vi "lab1_byte_packet_transceiver.vi"() -> ()   [LabVIEW 2014]
uses:
  <vilib>/addons/Modulation/Analog/controls/Complex Data Waveform.ctl
  <vilib>/addons/Modulation/Analog/support/mod_Set Error Source.vi
  <vilib>/addons/Modulation/Digital/Support/Common/Validators/mod_AWGN Validate.vi
  <vilib>/addons/Modulation/Digital/Impairments/subVIs/mod_createSeeds.vi
  <vilib>/addons/Modulation/Digital/Support/Common/Validators/mod_Validate Samples Per Symbol.vi
  <vilib>/addons/Modulation/Analog/support/Validators/mod_Validate Complex Waveform.vi
  <vilib>/addons/Modulation/Analog/support/Validators/mod_WFErrorHandler.vi
  <vilib>/addons/Modulation/Digital/General/MT Generate PSK System Parameters(M).vi
  <vilib>/addons/Modulation/Digital/Support/Common/Validators/mod_Generate Filter Coefficients Validate.vi
  <vilib>/addons/Modulation/Digital/General/subVIs/mod_Generate Filter Coefficients.vi
  <vilib>/addons/Modulation/Digital/General/subVIs/mod_Generate Bits PN Sequence.vi
  <vilib>/Analysis/1siggen.llb/Gaussian White Noise (obs 90).vi
  <vilib>/addons/Modulation/niDMT.lvlib
  <vilib>/addons/Modulation/niAMT.lvlib
panel:
  out "packet counter":u32
  in  "Eb/N0 (10 dB)":dbl=10.0 format="%.2f"
  out "Constellation Graph":T1(graph)
  in  "filter length (symbols)":i32=8
  in  "filter parameter":dbl=0.5 format="%.2f"
  in  "pulse shaping filter (none)":T2(ring)
  in  "M-PSK (4)":i32=4
  in  "samples per symbol (16)":i32=16
  out "rx history":string
  out "tx history":string
  out "rx instant":string
  out "found?":bool
  out "byte length":u32
  in  "OK Button":bool
  in  "stop":bool
  out "size(s)":i32
  in  "tx instant":string
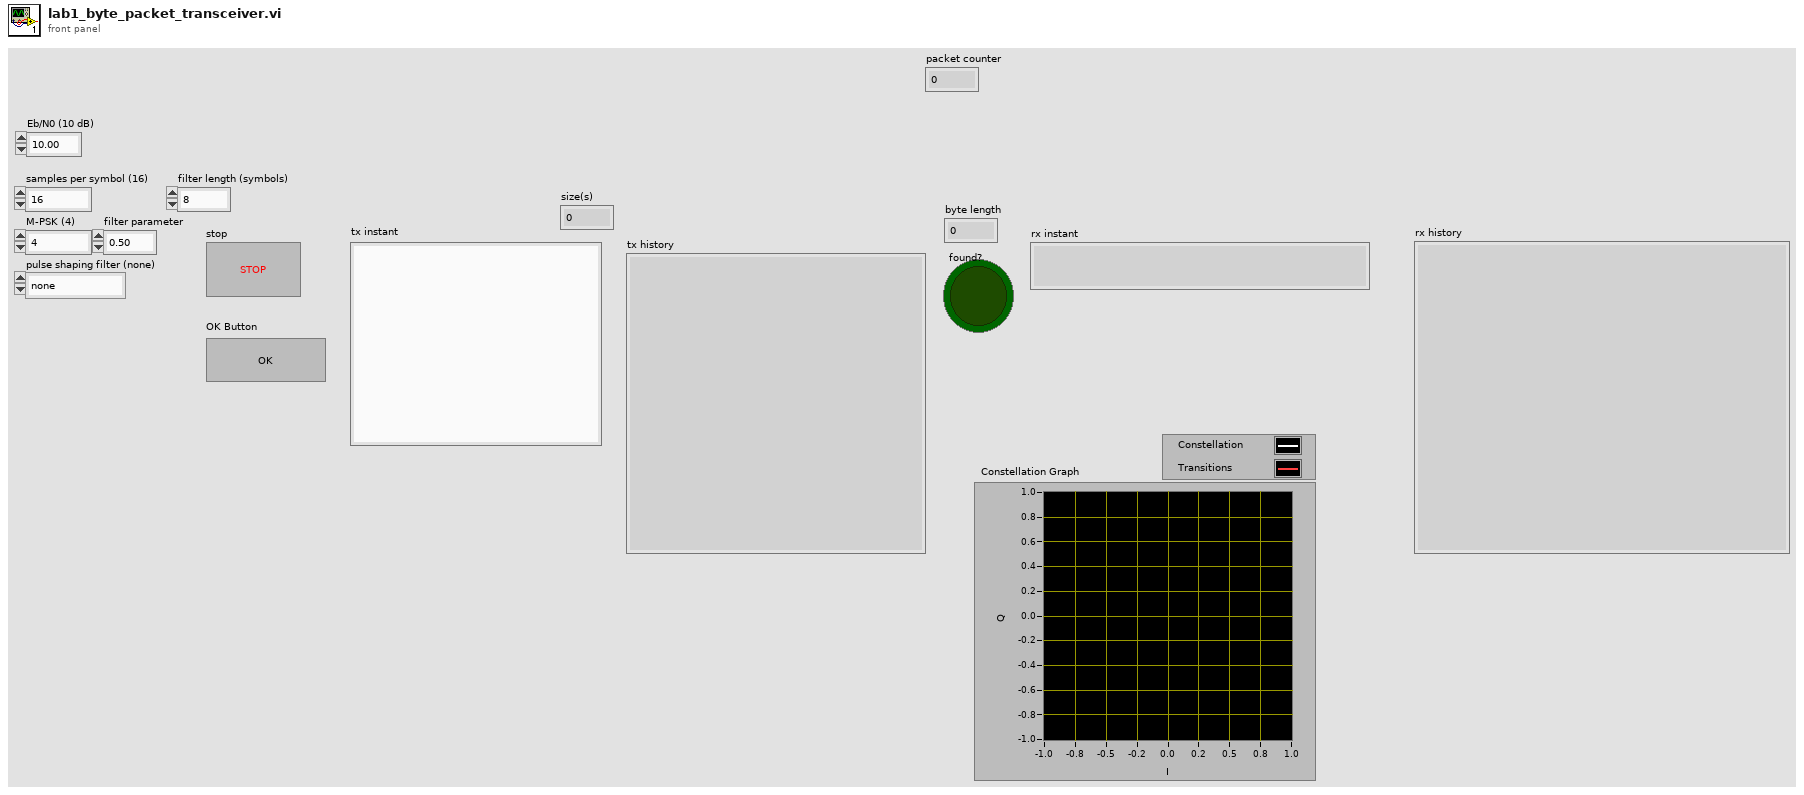
[diagram p1: front panel]
types:
  T1 = cluster{"Decimated Array":dbl[], "Decimated Array":dbl[]}[]
  T2 = enum16{"none", "Raised Cosine", "Root Raised Cos", "Gaussian"}
  T3 = typedef "niAMT.lvlib/Complex Data Waveform.ctl" = cluster{"t0":dbl, "dt":dbl, "Y":cdb[]}
  T4 = enum16{"FSK", "PSK", "QAM", "MSK", "PAM", "ASK", "CPM"}
  T5 = cluster{"samples per symbol (16)":i32, "symbol map":cdb[], "differential PSK":enum16{"disable", "enable"}, "PSK type":u16}
  T6 = cluster{"constellation":dbl[], "oversampled data":dbl[]}[]
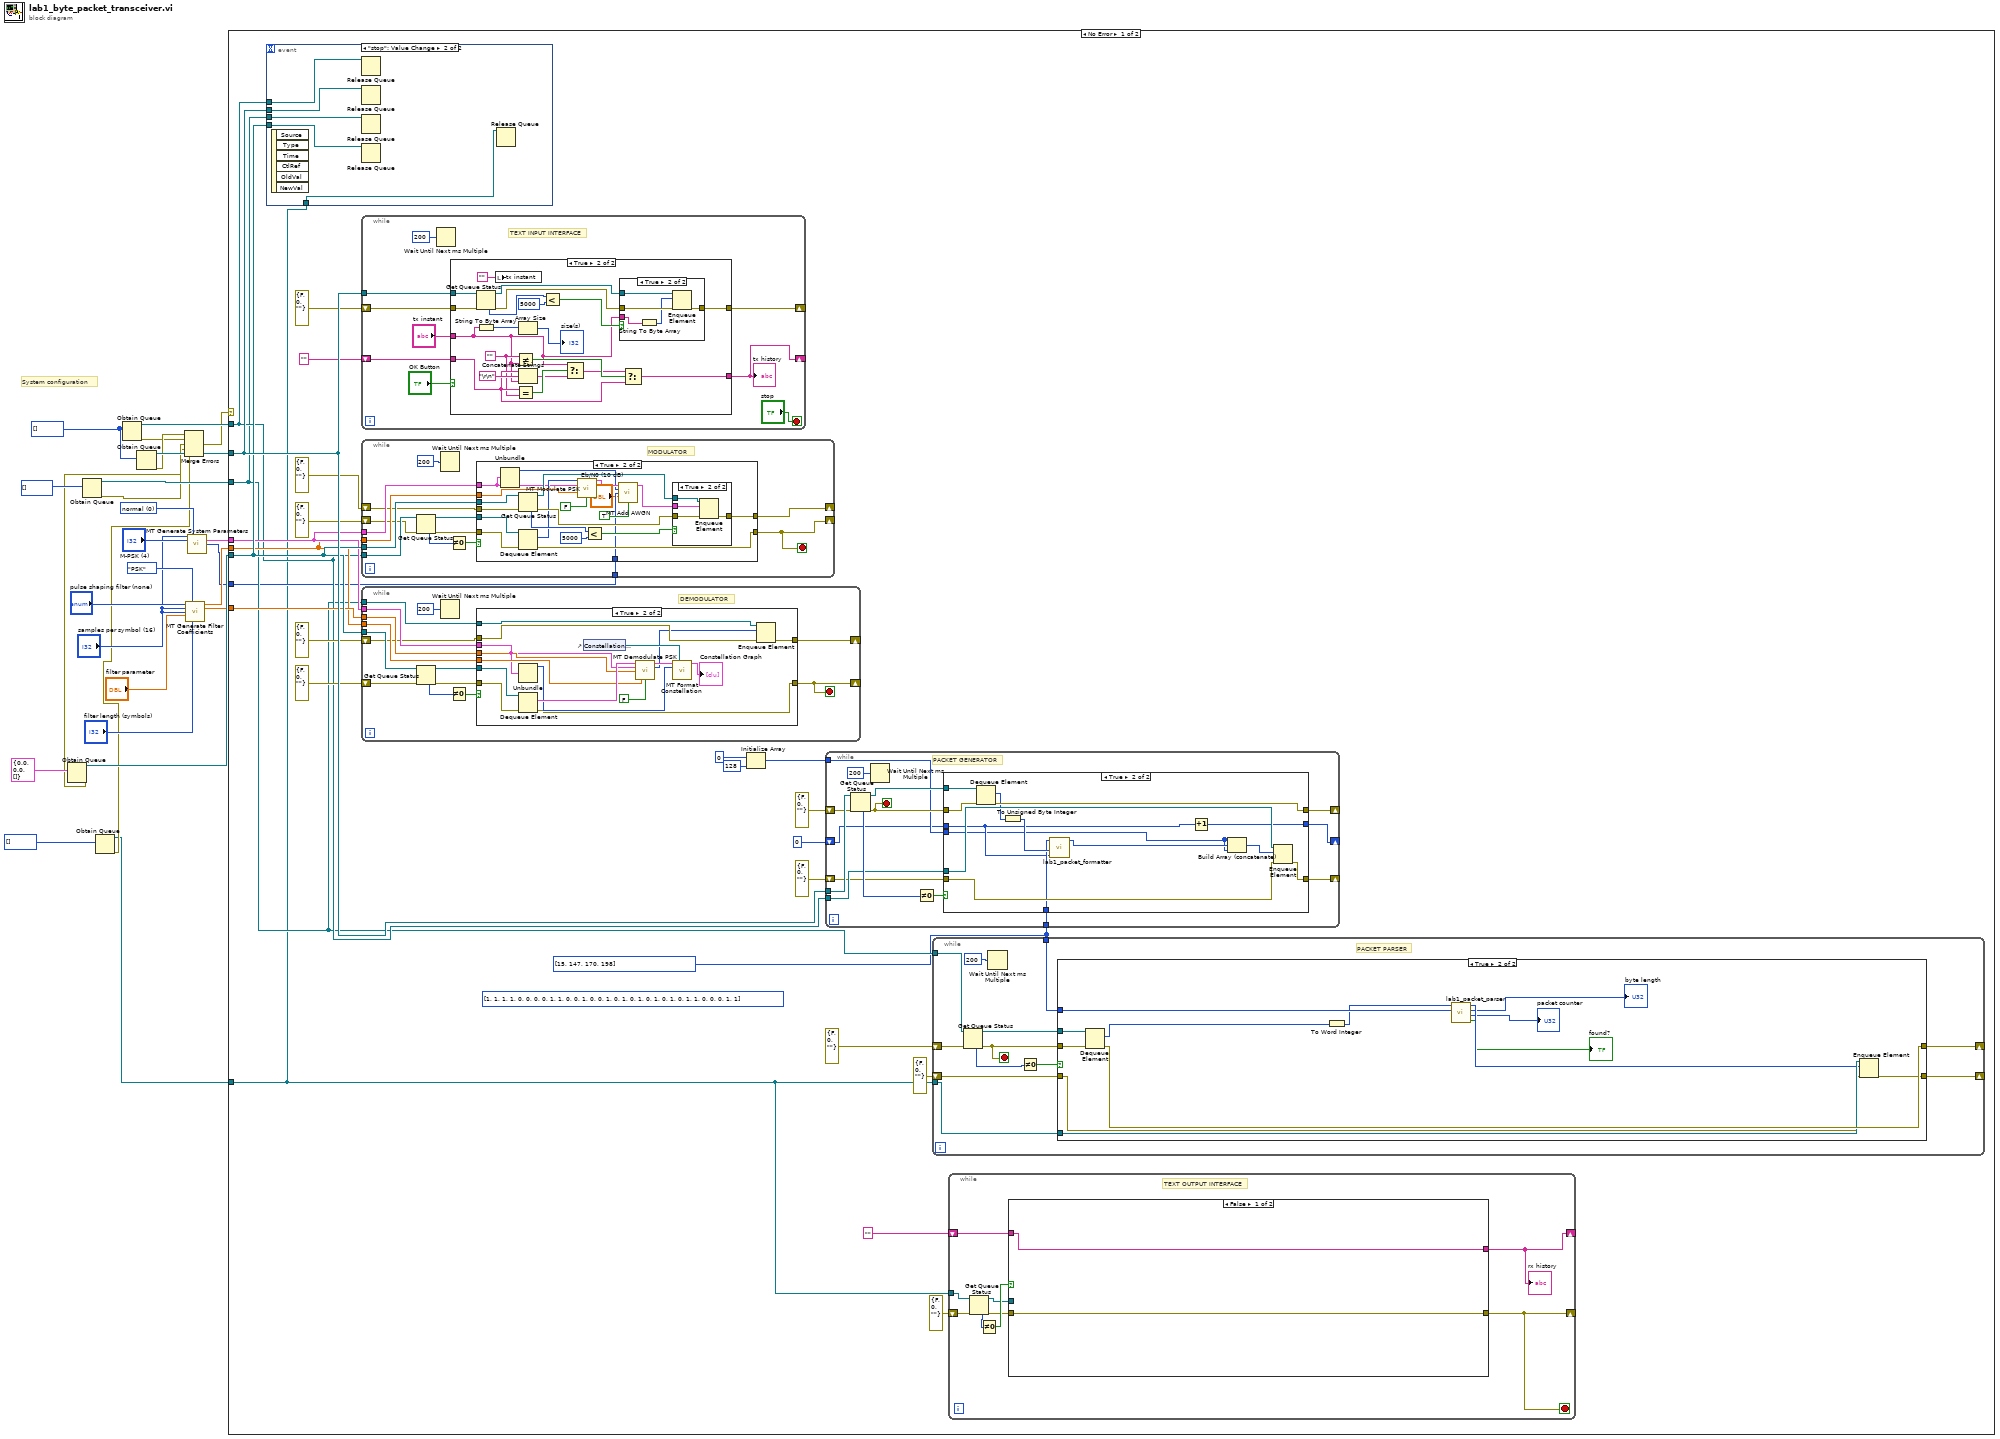
[diagram p0: block diagram]
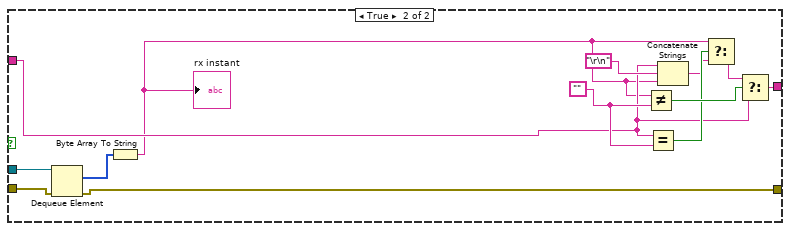
[diagram p2: hidden frame]
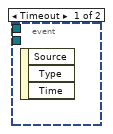
[diagram p7: hidden frame]
diagram:
  w21 = u16 0 items=["normal", "shifted", "offset"] ("PSK type")
  w7 = i32[] []
  # "System configuration"
  n1 = Obtain Queue(element data type=T3 {"t0"=0.0, "dt"=0.0, "Y"=[]} ("output complex waveform")) -> (queue out=w11:refnum<queue>, error out=w4:errorcluster)  [unwired: 4 in, 1 out]
  n2 = Obtain Queue(element data type=i32[] []) -> (queue out=w8:refnum<queue>, error out=w5:errorcluster)  [unwired: 4 in, 1 out]
  n3 = Obtain Queue(element data type=u8[] []) -> (queue out=w1:refnum<queue>, error out=w2:errorcluster)  [unwired: 4 in, 1 out]
  n4 = Obtain Queue(element data type=w7) -> (queue out=w23:refnum<queue>, error out=w24:errorcluster)  [unwired: 4 in, 1 out]
  n5 = Obtain Queue(element data type=w7) -> (queue out=w26:refnum<queue>, error out=w25:errorcluster)  [unwired: 4 in, 1 out]
  n6 = Merge Errors(w25, w24, w5, w4, w2) -> (w22:errorcluster)
  n7 = call <vilib>:"MT Generate Filter Coefficients.vi"("pulse shaping filter (none)"="pulse shaping filter (none)", "modulation type"=T4."PSK", "pulse shaping samples per symbol (16)"="samples per symbol (16)", "matched samples per symbol (16)"="samples per symbol (16)", "filter parameter"="filter parameter", "filter length (symbols)"="filter length (symbols)") -> ("pulse shaping filter coefficients"=w13:dbl[], "matched filter coefficients"=w10:dbl[])  [unwired: 7 in, 1 out]
  n8 = call-poly <vilib>:"MT Generate System Parameters.vi"("samples per symbol (16)"="samples per symbol (16)", "PSK type"=w21, "M-PSK (4)"="M-PSK (4)") -> ("PSK system parameters"=w14:T5, "bits per symbol"=w6:i32)  [unwired: 10 in, 1 out]
  n9 = case shown="No Error" w22 {
    tunnel: w26 -> [w51 _]
    tunnel: w23 -> [w39 _]
    tunnel: w14 -> [w44 _]
    tunnel: w13 -> [w42 _]
    tunnel: w11 -> [w45 _]
    tunnel: w10 -> [w43 _]
    tunnel: w8 -> [w37 _]
    tunnel: w6 -> [w33 _]
    tunnel: w1 -> [w28 _]
    frame No Error {
      w27 = u8[] [15, 147, 170, 198] ("Array")
      (unwired) i32[] [1, 1, 1, 1, 0, 0, 0, 0, 1, 1, 0, 0, 1, 0, 0, 1, 0, 1, 0, 1, 0, 1, 0, 1, 0, 1, 1, 0, 0, 0, 1, 1]
      n10 = event shown="[1] \"stop\": Value Change" {
        selector: _ -> [_ _]
        dyn-events: _ -> [_ _]
        timeout: _ -> [_ _]
        tunnel: w51 -> [_ w182]
        tunnel: w39 -> [_ w181]
        tunnel: w45 -> [_ w180]
        tunnel: w37 -> [_ w179]
        tunnel: w28 -> [_ w178]
        event Timeout {
          n11 = event-data() -> ()  [unwired: 1 in, 3 out]
        }
        event "stop": Value Change {
          n12 = event-data() -> ()  [unwired: 1 in, 6 out]
          n13 = Release Queue(queue=w181) -> ()  [unwired: 2 in, 3 out]
          n14 = Release Queue(queue=w182) -> ()  [unwired: 2 in, 3 out]
          n15 = Release Queue(queue=w179) -> ()  [unwired: 2 in, 3 out]
          n16 = Release Queue(queue=w180) -> ()  [unwired: 2 in, 3 out]
          n17 = Release Queue(queue=w178) -> ()  [unwired: 2 in, 3 out]
        }
      }
      n18 = while {
        tunnel: w51 -> [w219]
        shift-right: [w217] -> _
        shift-left: errorcluster {"status"=FALSE, "code"=0, "source"=""} ("error out") -> [w218]
        shift-right: [w215] -> _
        shift-left: "" -> [w216]
        stop <- "stop" stop-if-true
        # "TEXT INPUT INTERFACE"
        n19 = Wait Until Next ms Multiple(millisecond multiple=u32 200) -> ()  [unwired: 1 out]
        n20 = case shown="True" "OK Button" {
          tunnel: "tx instant" -> [_ w227]
          tunnel: w219 -> [_ w242]
          tunnel: w218 -> [w225 w236]
          tunnel: [w225 w235] -> w217
          tunnel: w216 -> [w224 w231]
          tunnel: [w224 w232] -> w215
          frame False {
          }
          frame True {
            w230 = ""
            n21 = Get Queue Status(queue=w242, error in (no error)=w236) -> (queue out=w238:refnum<queue>, error out=w237:errorcluster, # elements in queue=w241:i32)  [unwired: 1 in, 5 out]
            n22 = String To Byte Array(string=w227) -> (unsigned byte array=w244:u8[])
            n23 = local write "tx instant"("") -> ()
            n24 = Not Equal?(x=w230, y=w227) -> (x != y?=w233:bool)
            n25 = Equal?(x=w231, y=w230) -> (x = y?=w229:bool)
            n26 = Array Size(array=w244) -> (size(s)=→"size(s)":i32)
            n27 = Concatenate Strings(w231, "\r\n", w227) -> (w228:string)
            n28 = Less?(x=w241, y=5000) -> (x < y?=w239:bool)
            n29 = Select(t=w227, s=w229, f=w228) -> (s? t:f=w226:string)
            n30 = case shown="True" w239 {
              tunnel: w238 -> [_ w251]
              tunnel: w227 -> [_ w248]
              tunnel: w237 -> [w246 w250]
              tunnel: [w246 w249] -> w235
              frame False {
              }
              frame True {
                n31 = String To Byte Array(string=w248) -> (unsigned byte array=w247:u8[])
                n32 = Enqueue Element(queue=w251, element=w247, error in (no error)=w250) -> (error out=w249:errorcluster)  [unwired: 1 in, 2 out]
              }
            }
            n33 = Select(t=w226, s=w233, f=w231) -> (s? t:f=w232:string)
          }
        }
        "tx history" <- w215
      }
      n34 = while {
        tunnel: w44 -> [w122]
        tunnel: w42 -> [w121]
        tunnel: w45 -> [w120]
        shift-right: [w118] -> _
        shift-left: errorcluster {"status"=FALSE, "code"=0, "source"=""} ("error out") -> [w119]
        tunnel: w39 -> [w117]
        shift-right: [w110] -> _
        shift-left: errorcluster {"status"=FALSE, "code"=0, "source"=""} ("error out") -> [w112]
        tunnel: w33 -> [w109]
        stop <- w110 stop-if-true
        # "MODULATOR"
        n35 = Get Queue Status(queue=w117, error in (no error)=w112) -> (queue out=w113:refnum<queue>, error out=w114:errorcluster, # elements in queue=w116:i32)  [unwired: 1 in, 5 out]
        n36 = Wait Until Next ms Multiple(millisecond multiple=u32 200) -> ()  [unwired: 1 out]
        n37 = Not Equal To 0?(x=w116) -> (x != 0?=w115:bool)
        n38 = case shown="True" w115 {
          tunnel: w122 -> [_ w129]
          tunnel: w121 -> [_ w144]
          tunnel: w120 -> [_ w143]
          tunnel: w119 -> [w123 w137]
          tunnel: [w123 w136] -> w118
          tunnel: w114 -> [w124 w134]
          tunnel: w113 -> [_ w135]
          tunnel: [w124 w132] -> w110
          tunnel: w109 -> [_ w127]
          frame False {
          }
          frame True {
            n39 = Unbundle(w129) -> ("samples per symbol (16)"=w128:i32)  [unwired: 3 out]
            n40 = Get Queue Status(queue=w143, error in (no error)=w137) -> (queue out=w139:refnum<queue>, error out=w138:errorcluster, # elements in queue=w142:i32)  [unwired: 1 in, 5 out]
            n41 = Dequeue Element(queue=w135, error in (no error)=w134) -> (element=w133:i32[], error out=w132:errorcluster)  [unwired: 1 in, 2 out]
            n42 = call <vilib>:"MT Modulate PSK.vi"("input bit stream"=w133, "PSK system parameters"=w129, "pulse shaping filter coefficients"=w144, "reset? (T)"=FALSE) -> ("output complex waveform"=w130:T3)  [unwired: 9 in, 2 out]
            n43 = Less?(x=w142, y=5000) -> (x < y?=w140:bool)
            n44 = call <vilib>:"MT Add AWGN.vi"("input complex waveform"=w130, "samples per symbol (16)"=w128, "bits per symbol (1)"=w127, "Eb/N0 (10 dB)"="Eb/N0 (10 dB)", "reset? (T)"=TRUE) -> ("output complex waveform"=w125:T3)  [unwired: 8 in, 2 out]
            n45 = case shown="True" w140 {
              tunnel: w139 -> [_ w150]
              tunnel: w138 -> [w146 w149]
              tunnel: w125 -> [_ w148]
              tunnel: [w146 w147] -> w136
              frame False {
              }
              frame True {
                n46 = Enqueue Element(queue=w150, element=w148, error in (no error)=w149) -> (error out=w147:errorcluster)  [unwired: 1 in, 2 out]
              }
            }
          }
        }
      }
      n47 = while {
        tunnel: w45 -> [w90]
        shift-right: [w81] -> _
        shift-left: errorcluster {"status"=FALSE, "code"=0, "source"=""} ("error out") -> [w86]
        tunnel: w44 -> [w84]
        tunnel: w43 -> [w83]
        tunnel: w42 -> [w82]
        tunnel: w37 -> [w80]
        shift-right: [w79] -> _
        shift-left: errorcluster {"status"=FALSE, "code"=0, "source"=""} ("error out") -> [w78]
        stop <- w81 stop-if-true
        # "DEMODULATOR"
        n48 = Get Queue Status(queue=w90, error in (no error)=w86) -> (queue out=w87:refnum<queue>, error out=w85:errorcluster, # elements in queue=w89:i32)  [unwired: 1 in, 5 out]
        n49 = Wait Until Next ms Multiple(millisecond multiple=u32 200) -> ()  [unwired: 1 out]
        n50 = Not Equal To 0?(x=w89) -> (x != 0?=w88:bool)
        n51 = case shown="True" w88 {
          tunnel: w87 -> [_ w108]
          tunnel: w85 -> [w92 w107]
          tunnel: w84 -> [_ w99]
          tunnel: w83 -> [_ w105]
          tunnel: w82 -> [_ w104]
          tunnel: [w92 w97] -> w81
          tunnel: w80 -> [_ w96]
          tunnel: [w91 w95] -> w79
          tunnel: w78 -> [w91 w94]
          frame False {
          }
          frame True {
            n52 = Unbundle(w99) -> ("samples per symbol (16)"=w98:i32)  [unwired: 3 out]
            n53 = Dequeue Element(queue=w108, error in (no error)=w107) -> (element=w106:T3, error out=w97:errorcluster)  [unwired: 1 in, 2 out]
            n54 = control-ref of="Constellation Graph"() -> (w101:refnum<vi>)
            n55 = call <vilib>:"MT Demodulate PSK.vi"("input complex waveform"=w106, "PSK system parameters"=w99, "matched filter coefficients"=w105, "pulse shaping filter coefficients"=w104, "reset? (T)"=FALSE) -> ("recovered complex waveform"=w100:T3, "output bit stream"=w93:i8[])  [unwired: 6 in, 3 out]
            n56 = call <vilib>:"MT Format Constellation.vi"("waveform"=w100, "constellation reference"=w101, "samples per symbol"=w98) -> ("constellation graph"=→"Constellation Graph":T6)  [unwired: 2 in, 10 out]
            n57 = Enqueue Element(queue=w96, element=w93, error in (no error)=w94) -> (error out=w95:errorcluster)  [unwired: 1 in, 2 out]
          }
        }
      }
      n58 = Initialize Array(0, 128 ("dimension size")) -> (w34:i32[])
      n59 = while {
        tunnel: w51 -> [w197]
        shift-right: [w191] -> _
        shift-left: errorcluster {"status"=FALSE, "code"=0, "source"=""} ("error out") -> [w196]
        tunnel: w39 -> [w189]
        shift-right: [w187] -> _
        shift-left: errorcluster {"status"=FALSE, "code"=0, "source"=""} ("error out") -> [w188]
        tunnel: w34 -> [w186]
        tunnel: w27 -> [w185]
        shift-right: [w183] -> _
        shift-left: 0 -> [w184]
        stop <- w192 stop-if-true
        # "PACKET GENERATOR"
        n60 = Get Queue Status(queue=w197, error in (no error)=w196) -> (queue out=w193:refnum<queue>, error out=w192:errorcluster, # elements in queue=w195:i32)  [unwired: 1 in, 5 out]
        n61 = Wait Until Next ms Multiple(millisecond multiple=u32 200) -> ()  [unwired: 1 out]
        n62 = Not Equal To 0?(x=w195) -> (x != 0?=w194:bool)
        n63 = case shown="True" w194 {
          tunnel: w193 -> [_ w214]
          tunnel: w192 -> [w200 w213]
          tunnel: [w200 w212] -> w191
          tunnel: w189 -> [_ w211]
          tunnel: w188 -> [w199 w210]
          tunnel: [w199 w209] -> w187
          tunnel: w186 -> [_ w201]
          tunnel: w185 -> [_ w205]
          tunnel: w184 -> [w198 w203]
          tunnel: [w198 w204] -> w183
          frame False {
          }
          frame True {
            n64 = Dequeue Element(queue=w214, error in (no error)=w213) -> (element=w207:i32[], error out=w212:errorcluster)  [unwired: 1 in, 2 out]
            n65 = To Unsigned Byte Integer(number=w207) -> (unsigned 8bit integer=w206:u8[])
            n66 = call "lab1_packet_formatter.vi"("counter"=w203, "payload(bytes array)"=w206, "preamble(bytes array)"=w205) -> ("bitstream"=w202:i16[])  [unwired: 8 in]
            n67 = Increment(x=w203) -> (x+1=w204:i32)
            n68 = Build Array (concatenate)(w201, w202, w201) -> (w208:i32[])
            n69 = Enqueue Element(queue=w211, element=w208, error in (no error)=w210) -> (error out=w209:errorcluster)  [unwired: 1 in, 2 out]
          }
        }
      }
      n70 = while {
        tunnel: w37 -> [w162]
        shift-right: [w155] -> _
        shift-left: errorcluster {"status"=FALSE, "code"=0, "source"=""} ("error out") -> [w160]
        tunnel: w28 -> [w154]
        shift-right: [w153] -> _
        shift-left: errorcluster {"status"=FALSE, "code"=0, "source"=""} ("error out") -> [w152]
        tunnel: w27 -> [w151]
        stop <- w156 stop-if-true
        # "PACKET PARSER"
        n71 = Get Queue Status(queue=w162, error in (no error)=w160) -> (queue out=w157:refnum<queue>, error out=w156:errorcluster, # elements in queue=w159:i32)  [unwired: 1 in, 5 out]
        n72 = Wait Until Next ms Multiple(millisecond multiple=u32 200) -> ()  [unwired: 1 out]
        n73 = Not Equal To 0?(x=w159) -> (x != 0?=w158:bool)
        n74 = case shown="True" w158 {
          tunnel: w157 -> [_ w177]
          tunnel: w156 -> [w164 w176]
          tunnel: [w164 w175] -> w155
          tunnel: w154 -> [_ w174]
          tunnel: [w163 w173] -> w153
          tunnel: w152 -> [w163 w172]
          tunnel: w151 -> [_ w171]
          frame False {
          }
          frame True {
            n75 = Dequeue Element(queue=w177, error in (no error)=w176) -> (element=w170:i32[], error out=w175:errorcluster)  [unwired: 1 in, 2 out]
            n76 = To Word Integer(number=w170) -> (16bit integer=w169:i16[])
            n77 = call "lab1_packet_parser.vi"("preamble bytes"=w171, "bitstream"=w169) -> ("Found?"=→"found?":bool, "packet counter"=→"packet counter":u32, "payload length(bytes)"=→"byte length":u32, "payload bytes"=w168:u8[])  [unwired: 6 in]
            n78 = Enqueue Element(queue=w174, element=w168, error in (no error)=w172) -> (error out=w173:errorcluster)  [unwired: 1 in, 2 out]
          }
        }
      }
      n79 = while {
        shift-right: [w60] -> _
        shift-left: "" -> [w61]
        tunnel: w28 -> [w59]
        shift-right: [w53] -> _
        shift-left: errorcluster {"status"=FALSE, "code"=0, "source"=""} ("error out") -> [w54]
        stop <- w53 stop-if-true
        # "TEXT OUTPUT INTERFACE"
        n80 = Get Queue Status(queue=w59, error in (no error)=w54) -> (queue out=w56:refnum<queue>, error out=w55:errorcluster, # elements in queue=w58:i32)  [unwired: 1 in, 5 out]
        n81 = Not Equal To 0?(x=w58) -> (x != 0?=w57:bool)
        n82 = case shown="False" w57 {
          tunnel: w61 -> [w63 w65]
          tunnel: [w63 w72] -> w60
          tunnel: w56 -> [_ w71]
          tunnel: w55 -> [w62 w70]
          tunnel: [w62 w69] -> w53
          frame False {
          }
          frame True {
            w75 = ""
            n83 = Dequeue Element(queue=w71, error in (no error)=w70) -> (element=w68:u8[], error out=w69:errorcluster)  [unwired: 1 in, 2 out]
            n84 = Byte Array To String(unsigned byte array=w68) -> (string=w64:string)
            "rx instant" <- w64
            n85 = Not Equal?(x=w64, y=w75) -> (x != y?=w74:bool)
            n86 = Equal?(x=w65, y=w75) -> (x = y?=w73:bool)
            n87 = Concatenate Strings(w65, "\r\n", w64) -> (w66:string)
            n88 = Select(t=w64, s=w73, f=w66) -> (s? t:f=w67:string)
            n89 = Select(t=w67, s=w74, f=w65) -> (s? t:f=w72:string)
          }
        }
        "rx history" <- w60
      }
    }
    frame Error {
    }
  }
